vi "Write Return Notifier.vi"(8 "error in (no error)":errorcluster, 10 "Return Notifier":refnum<notifier>, 11 "Timing Engine Tester in":refnum<class "Timing Engine Tester.lvclass">) -> (0 "error out":errorcluster, 3 "Timing Engine Tester out":refnum<class "Timing Engine Tester.lvclass">)   [LabVIEW 2018, in "Timing Engine Tester.lvlib" / "Timing Engine Tester.lvclass"]
uses:
  Timing Engine Tester.lvclass
  Timing Engine Tester.lvclass/Timing Engine Tester.ctl
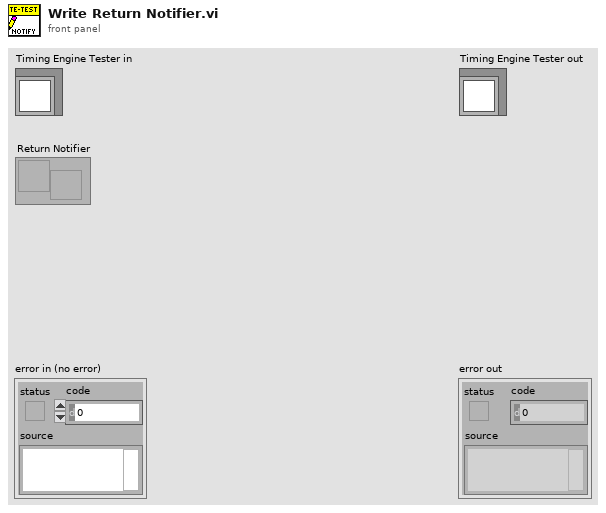
[diagram p1: front panel]
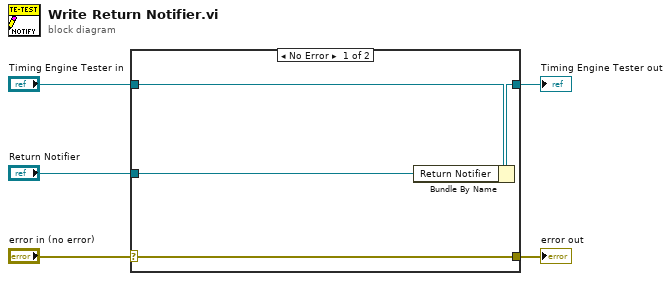
[diagram p0: block diagram]
diagram:
  n1 = case shown="No Error" "error in (no error)" {
    selector: "error in (no error)" -> [w9 w10]
    tunnel: [w9 w10] -> w4
    tunnel: [w7 w11] -> w2
    tunnel: "Timing Engine Tester in" -> [w8 w11]
    tunnel: "Return Notifier" -> [w6 _]
    frame No Error {
      n2 = Bundle By Name(cluster=w8, "Return Notifier"=w6) -> (w7:refnum<class "Timing Engine Tester.lvclass">)
    }
    frame Error {
    }
  }
  "error out" <- w4
  "Timing Engine Tester out" <- w2
